vi "CreateIterator.vi"(8 "error in (no error)":errorcluster, 11 "BrowerLeaf in":refnum<class "BrowerLeaf.lvclass">) -> (0 "error out":errorcluster, 2 "Iterator":refnum<class "Iterator.lvclass">, 3 "BrowerLeaf out":refnum<class "BrowerLeaf.lvclass">)   [LabVIEW 2015, in "BrowerLeaf.lvclass"]
uses:
  BrowerLeaf.lvclass
  Iterator/Interface/Iterator.lvclass
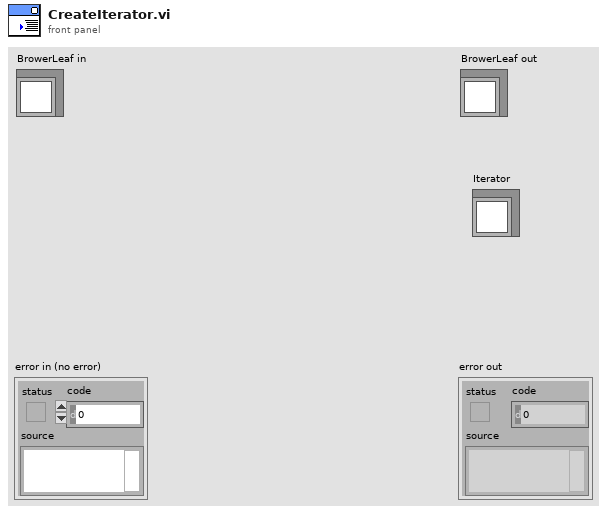
[diagram p1: front panel]
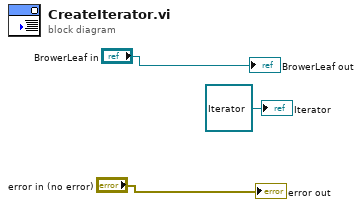
[diagram p0: block diagram]
diagram:
  "error out" <- "error in (no error)"
  "BrowerLeaf out" <- "BrowerLeaf in"
  "Iterator" <- refnum<class "Iterator.lvclass"> refnum ("Iterator")
